vi "Analyse.vi"(8 "error in (no error)":errorcluster, 10 "ImageData":T1, 11 "FluorescenceAnalyserNTU in":refnum<class "FluorescenceAnalyserNTU.lvclass">) -> (0 "error out":errorcluster, 3 "FluorescenceAnalyserNTU out":refnum<class "FluorescenceAnalyserNTU.lvclass">)   [LabVIEW 2011, in "Tools.lvlib" / "Imaging.lvlib" / "FluorescenceAnalyserNTU.lvclass"]
uses:
  FluorescenceAnalyserNTU.lvclass
  FluorescenceAnalyserNTU.lvclass/FluorescenceAnalyserNTU.ctl
  FluorescenceAnalyser/FluorescenceAnalyser.lvclass
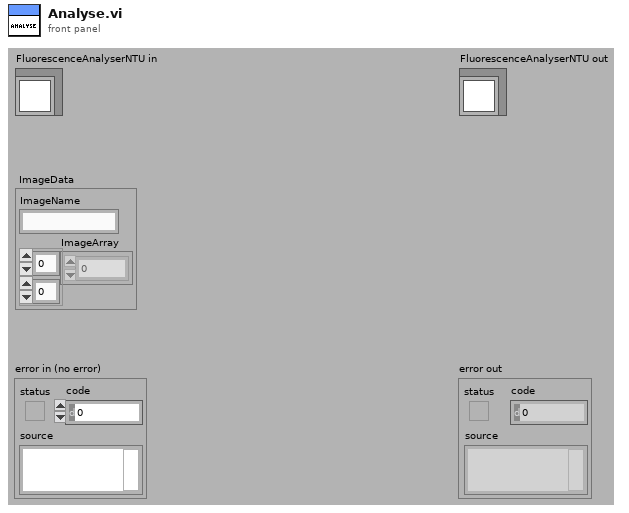
[diagram p1: front panel]
types:
  T1 = cluster{"ImageName":string, "ImageArray":sgl[][]}
  T2 = cluster{"ImageName":string, "ImageArray":sgl[][]}[]
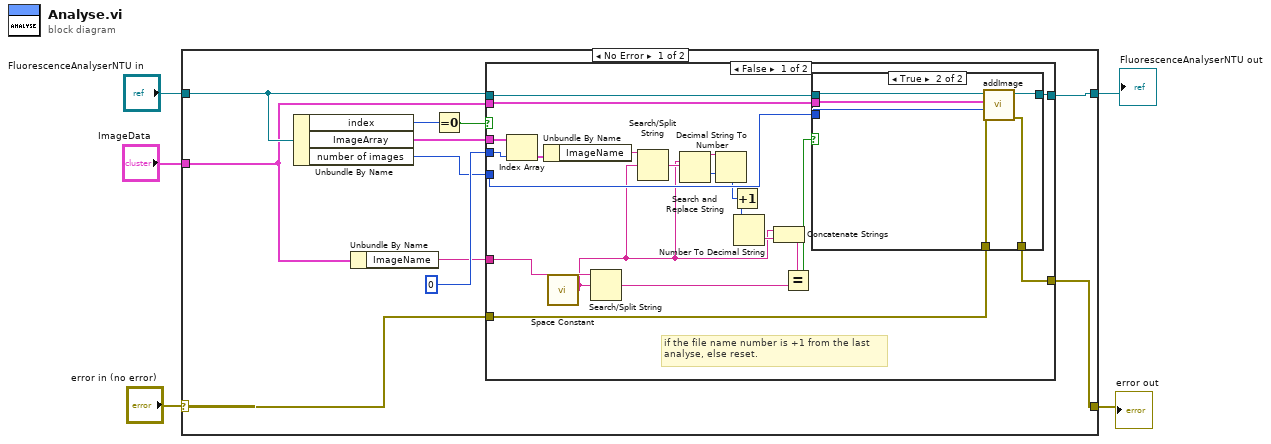
[diagram p0: block diagram]
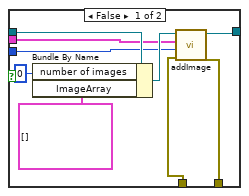
[diagram p2: hidden frame]
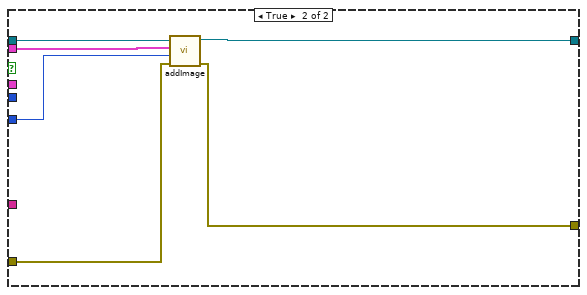
[diagram p3: hidden frame]
diagram:
  n1 = case shown="No Error" "error in (no error)" {
    selector: "error in (no error)" -> [w6 w59]
    tunnel: [w8 w59] -> w4
    tunnel: "FluorescenceAnalyserNTU in" -> [w10 w58]
    tunnel: [w9 w58] -> w2
    tunnel: "ImageData" -> [w7 _]
    frame No Error {
      n2 = Unbundle By Name(w10) -> ("index"=w13:i32, "ImageArray"=w16:T2, "number of images"=w11:i32)
      n3 = Unbundle By Name(w7) -> ("ImageName"=w12:string)
      n4 = Equal To 0?(x=w13) -> (x = 0?=w14:bool)
      n5 = case shown="False" w14 {
        tunnel: [w31 w57] -> w9
        tunnel: w6 -> [w29 w56]
        tunnel: [w28 w55] -> w8
        tunnel: w7 -> [w30 w54]
        tunnel: w10 -> [w32 w52]
        tunnel: w16 -> [w35 _]
        tunnel: 0 -> [w36 _]
        tunnel: w12 -> [w25 _]
        tunnel: w11 -> [w27 w53]
        frame False {
          # "if the file name number is +1 from the last\nanalyse, else reset."
          n6 = Index Array(array=w35, index=w36) -> (element=w34:T1)
          n7 = Unbundle By Name(w34) -> ("ImageName"=w26:string)
          n8 = call <vilib>:"Space Constant.vi"() -> ("String"=w18:string)
          n9 = Search/Split String(string=w25, search string/char (-)=w18) -> (match + rest of string=w17:string)  [unwired: 1 in, 2 out]
          n10 = Search/Split String(string=w26, search string/char (-)=w18) -> (match + rest of string=w24:string)  [unwired: 1 in, 2 out]
          n11 = Search and Replace String(input string=w24, search string=w18) -> (result string=w23:string, offset past replacement=w22:i32)  [unwired: 6 in, 2 out]
          n12 = Decimal String To Number(string=w23) -> ()  [unwired: 2 in, 2 out]
          n13 = Increment(x=w22) -> (x+1=w21:i32)
          n14 = Number To Decimal String(number=w21) -> (decimal integer string=w20:string)  [unwired: 1 in]
          n15 = Concatenate Strings(w18, w20) -> (w19:string)
          n16 = Equal?(x=w19, y=w17) -> (x = y?=w33:bool)
          n17 = case shown="True" w33 {
            tunnel: w32 -> [w44 w51]
            tunnel: [w37 w50] -> w31
            tunnel: w30 -> [w41 w49]
            tunnel: w29 -> [w39 w48]
            tunnel: [w38 w47] -> w28
            tunnel: w27 -> [w40 w46]
            frame False {
              n18 = Bundle By Name(cluster=w44, "number of images"=0, "ImageArray"=T2 []) -> (w42:refnum<class "FluorescenceAnalyserNTU.lvclass">)
              n19 = call "addImage.vi"("error in (no error)"=w39, "number of images"=w40, "ImageData"=w41, "FluorescenceAnalyser in"=w42) -> ("error out"=w38:errorcluster, "FluorescenceAnalyser out"=w37:refnum<class "FluorescenceAnalyserNTU.lvclass">)  [unwired: 6 in]
            }
            frame True {
              n20 = call "addImage.vi"("error in (no error)"=w48, "number of images"=w46, "ImageData"=w49, "FluorescenceAnalyser in"=w51) -> ("error out"=w47:errorcluster, "FluorescenceAnalyser out"=w50:refnum<class "FluorescenceAnalyserNTU.lvclass">)  [unwired: 6 in]
            }
          }
        }
        frame True {
          n21 = call "addImage.vi"("error in (no error)"=w56, "number of images"=w53, "ImageData"=w54, "FluorescenceAnalyser in"=w52) -> ("error out"=w55:errorcluster, "FluorescenceAnalyser out"=w57:refnum<class "FluorescenceAnalyserNTU.lvclass">)  [unwired: 6 in]
        }
      }
    }
    frame Error {
    }
  }
  "error out" <- w4
  "FluorescenceAnalyserNTU out" <- w2
